vi "Fetch Multi Eval Meas Trace Power Monitor Results.vi"(8 "error in (no error)":errorcluster, 10 "Instance (1)":T1=1, 11 "VISA resource name":refnum<visa-resource-name>) -> (0 "error out":errorcluster, 1 "Trace Power Monitor Results":dbl[](array[numeric]) format="%^.3e", 2 "Reliability":i32, 3 "VISA resource name out":refnum<visa-resource-name>)   [LabVIEW 2015, in "Rohde&Schwarz CMXP NR FR2 Measurement.lvlib"]
doc: "Returns the power monitor results.\n\nAttribute:\nRSCMXPNRFR2M_ATTR_FETCH_MULTI_EVAL_MEASUREMENT_TRACE_POWER_MONITOR_RESULTS\n\nRemote-control command:\nFETCh:NRMMw:MEAS<i>:MEValuation:TRACe:PMONitor?"
uses:
  <instrlib>/Rohde&Schwarz CMXP NR FR2 Measurement/Rohde&Schwarz CMXP NR FR2 Measurement.lvlib
  <instrlib>/Rohde&Schwarz CMXP NR FR2 Measurement/Private/_Instance.ctl
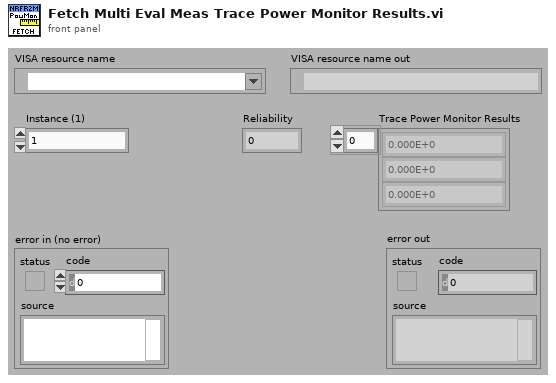
[diagram p1: front panel]
types:
  T1 = typedef "Rohde&Schwarz CMXP NR FR2 Measurement.lvlib/_Instance.ctl" = i32
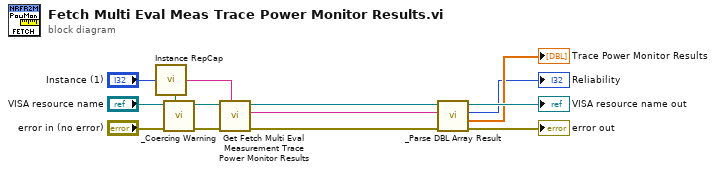
[diagram p0: block diagram]
diagram:
  n1 = call <instrlib>:"Instance RepCap.vi"("Instance In"="Instance (1)") -> ("In Range?"=w12:bool, "RepCap Identifier Out"=w9:string)  [unwired: 1 in]
  n2 = call <instrlib>:"_Coercing Warning.vi"("In Range?"=w12, "error in (no error)"="error in (no error)", "VISA resource name"="VISA resource name") -> ("error out"=w10:errorcluster, "VISA resource name out"=w11:refnum<visa-resource-name>)  [unwired: 7 in]
  n3 = call "Get Fetch Multi Eval Measurement Trace Power Monitor Results"("Repeated Capabilities"=w9, "error in (no error)"=w10, "instrument handle"=w11) -> ("error out"=w7:errorcluster, "Fetch Multi Eval Measurement Trace Power Monitor Results"=w6:string, "instrument handle out"=w8:refnum<visa-resource-name>)  [unwired: 6 in]
  n4 = call <instrlib>:"_Parse DBL Array Result.vi"("error in (no error)"=w7, "Input String"=w6, "VISA resource name"=w8) -> ("error out"=→"error out":errorcluster, "Results"=→"Trace Power Monitor Results":dbl[], "Reliability"=→"Reliability":i32, "VISA resource name out"=→"VISA resource name out":refnum<visa-resource-name>)  [unwired: 5 in]
